vi "探头窗口-20-服务器版.vi"() -> ()   [LabVIEW 2013]
panel:
  in  "外部停止命令？":bool=TRUE
  out "引用-探头属性[]":refnum<vi>
  out "引用-监测模式？":refnum<vi>
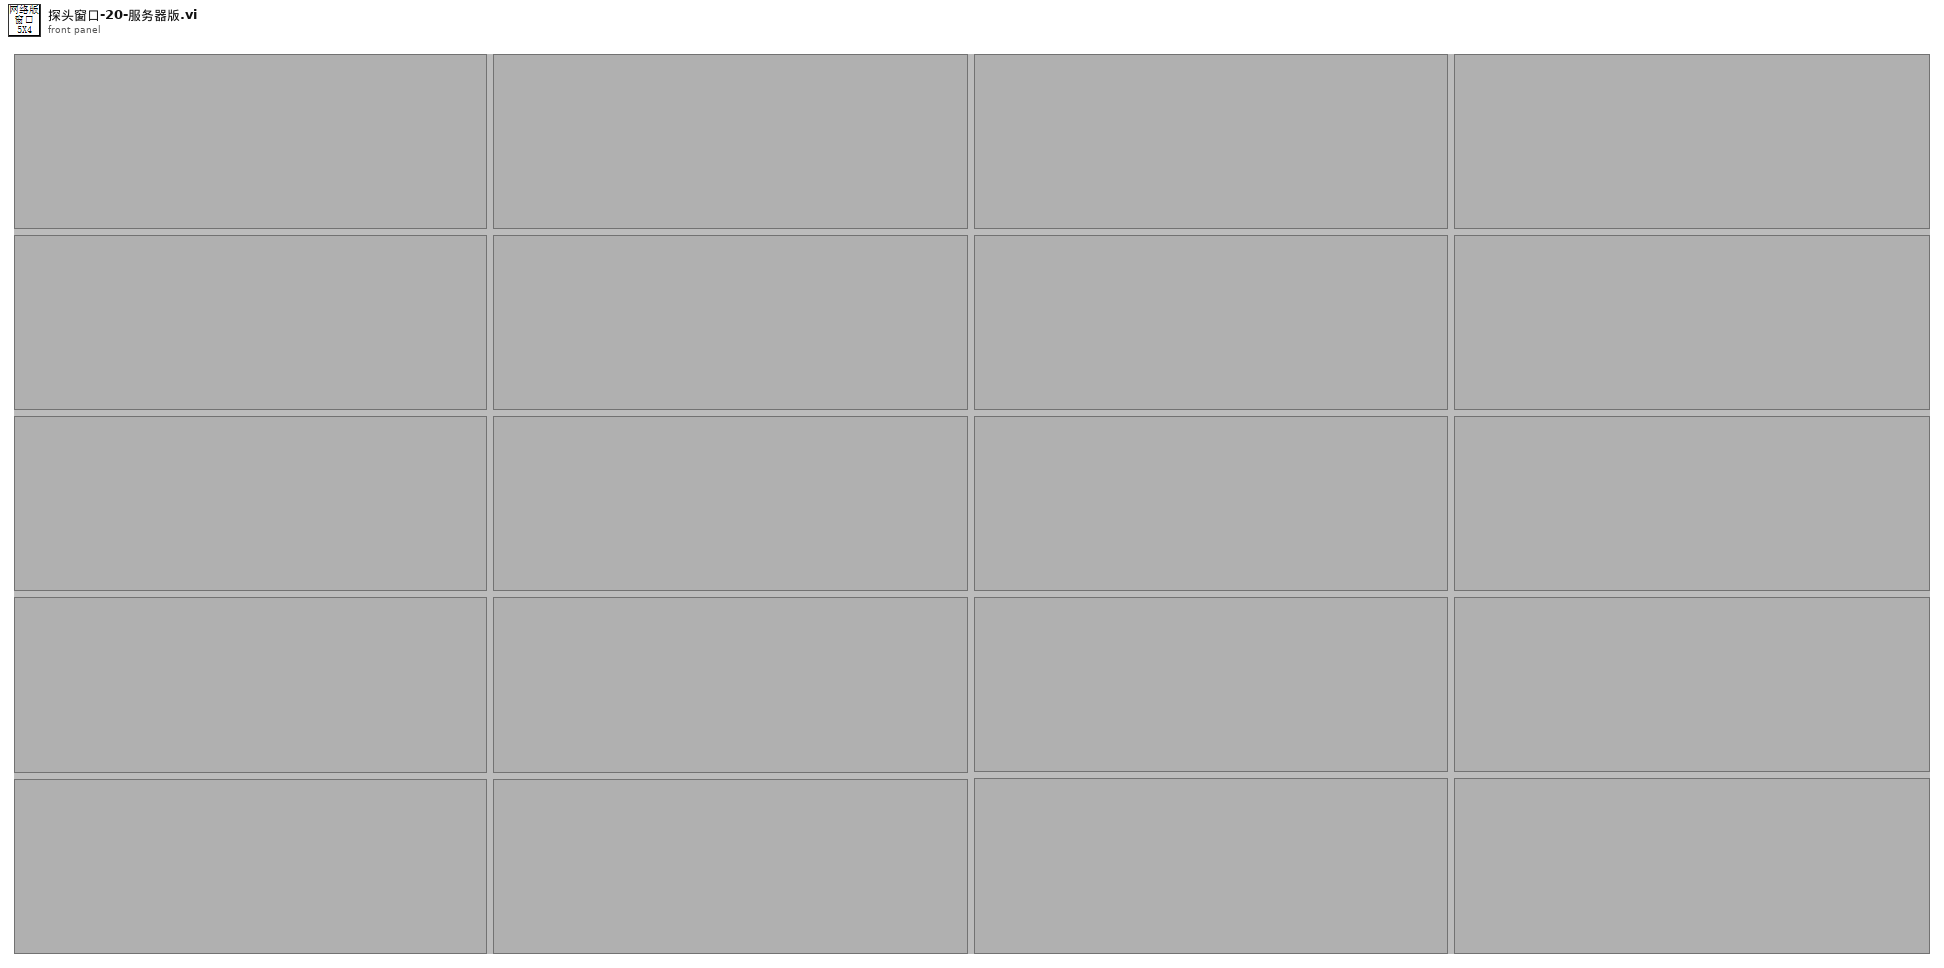
[diagram p1: front panel]
types:
  T1 = typedef "eventvkey.ctl" = enum16{"ASCII", "Enter", "Return", "Shift", "Ctrl", "Alt", "Cmd", "Opt", "Caps", "NumLock", "Clear", "Break", "Up", "Down", "Left", "Right", "Insert", "Delete", "Home", "End", "PageUp", "PageDown", "Escape", "Help", "Pause", "ScrollLock", "F1", "F2", "F3", "F4", "F5", "F6", "F7", "F8", "F9", "F10", "F11", "F12", "F13", "F14", "F15", "F16", "F17", "F18", "F19", "F20", "F21", "F22", "F23", "F24", "Play", "VolumeUp", "VolumeDown", "Mute", "Two Byte Char"}
  T2 = cluster{"探头地址与信息":cluster{"网络地址":cluster{"IP":string, "port":u16}, "探头信息":string}, "测量值":cluster{"时间":timestamp, "数值":dbl}, "限值":cluster{"限值1":dbl, "限值2":dbl}, "探头状态":enum16{"正常", "离线", "禁用", "一级报警", "二级报警"}}[]
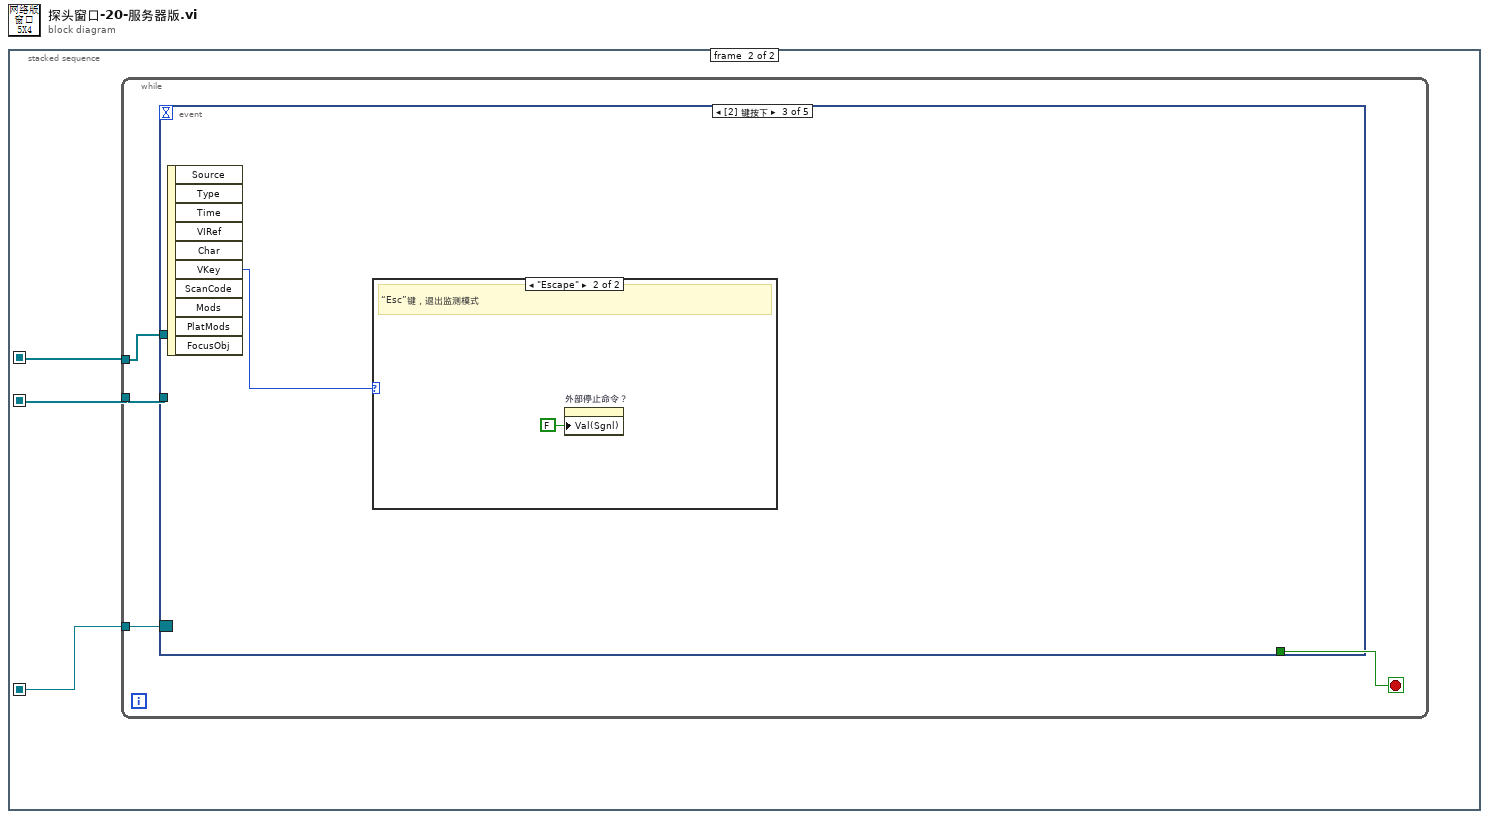
[diagram p0: block diagram]
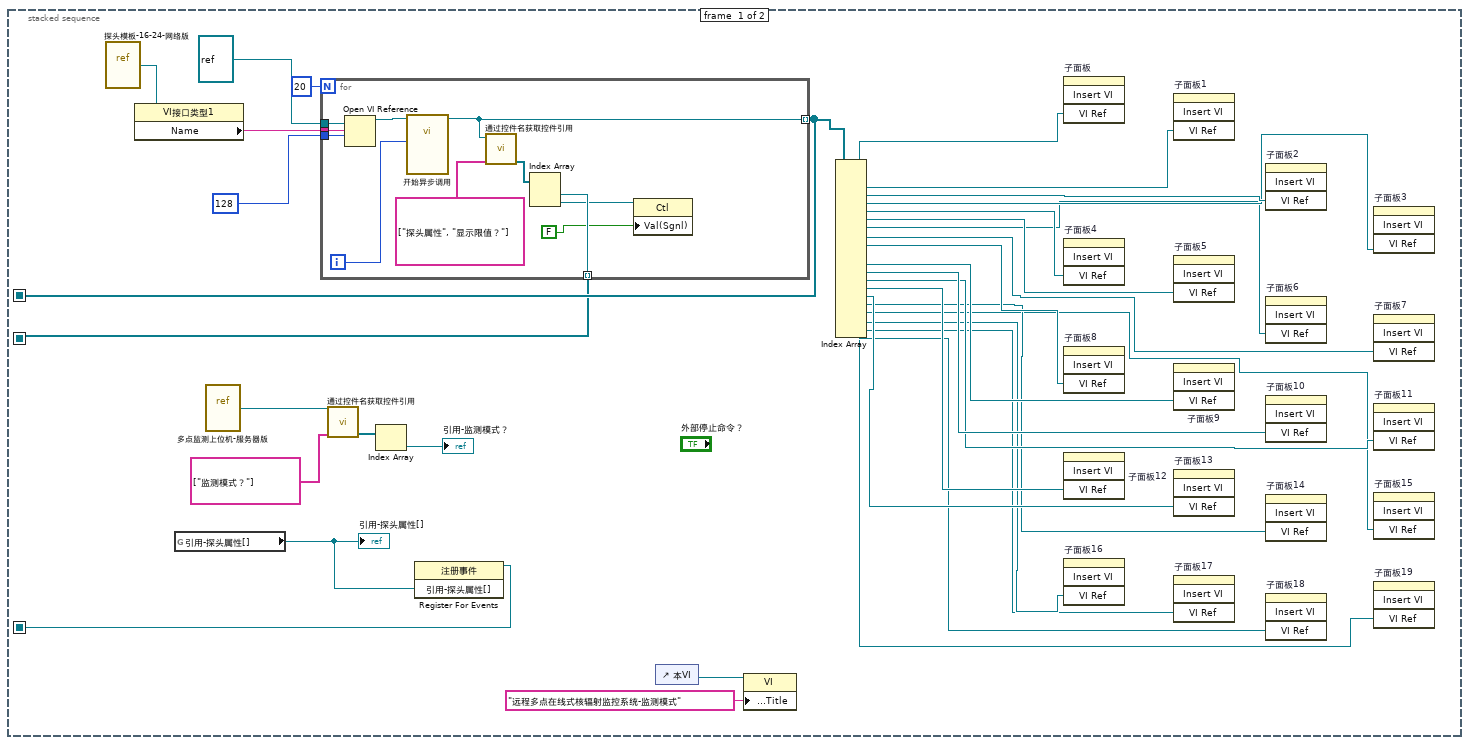
[diagram p2: hidden frame]
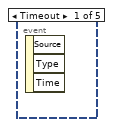
[diagram p3: hidden frame]
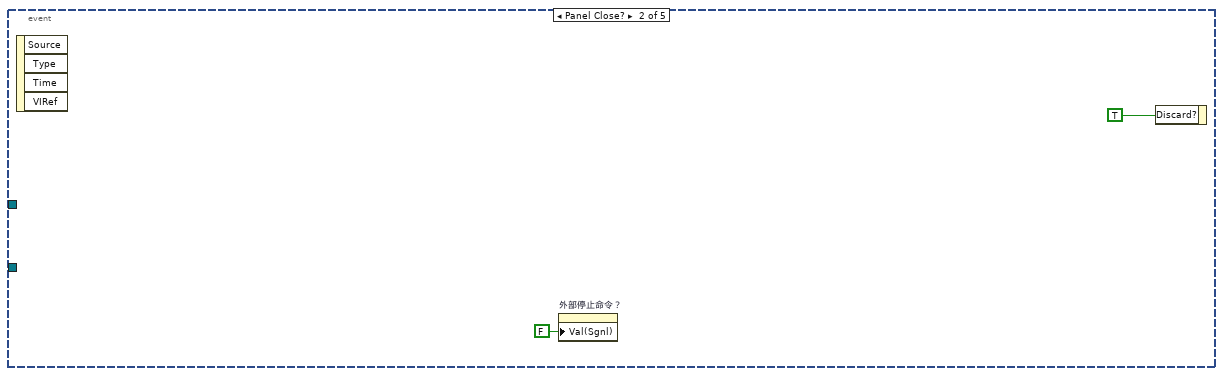
[diagram p4: hidden frame]
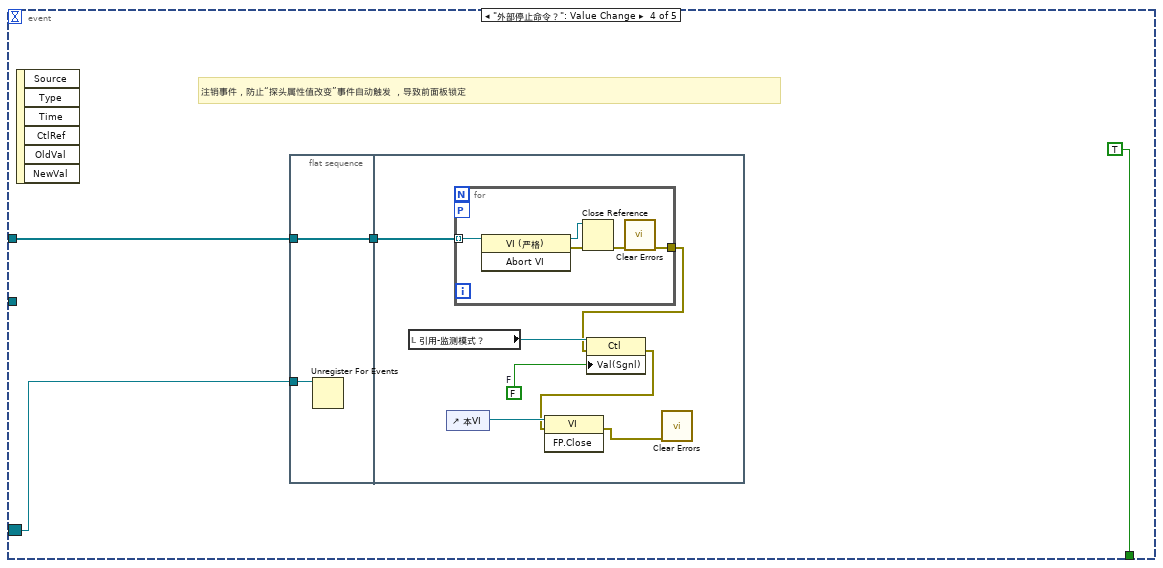
[diagram p6: hidden frame]
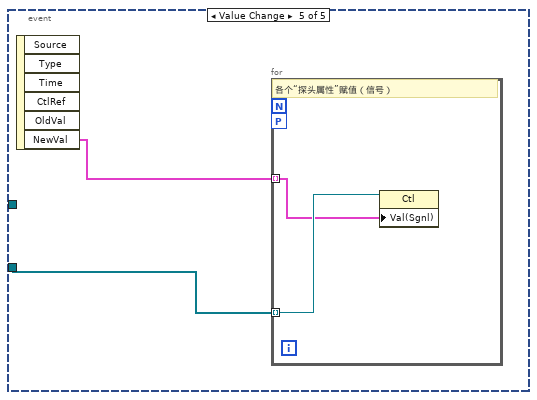
[diagram p7: hidden frame]
diagram:
  n1 = stacked-sequence {
    seq-local: [w30 _] -> [_ w49]
    seq-local: [w9 _] -> [_ w48]
    seq-local: [w3 _] -> [_ w47]
    frame #0 {
      n2 = vi-ref "探头模板-16-24-网络版.vi"() -> (w35:refnum<vi>)
      n3 = property class="VI接口类型1"(reference=w35) -> ("Name"=w34:string)  [unwired: 1 in, 2 out]
      n4 = global read "全局变量-35点监测.vi" "引用-探头属性[]"() -> (w4:refnum<vi>)
      "引用-探头属性[]" <- w4
      n5 = vi-ref "多点监测上位机-服务器版.vi"() -> (w5:refnum<vi>)
      n6 = for {
        N: 20 -> [_]
        tunnel: w34 -> [w46]
        tunnel: 128 ("选项") -> [w45]
        tunnel: refnum<vi> refnum ("类型说明符VI引用句柄（仅用于类型）") -> [w44]
        tunnel: [w39] -> w30 mode=indexing
        tunnel: [w40] -> w9 mode=indexing
        i -> [w36]
        n7 = Open VI Reference(type specifier VI Refnum (for type only)=w44, vi path=w46, options=w45) -> (vi reference=w41:refnum<vi>)  [unwired: 3 in, 1 out]
        n8 = call-by-ref "开始异步调用"(reference=w41, "探头序号"=w36) -> (reference out=w39:refnum<vi>)  [unwired: 12 in, 1 out]
        n9 = call "通过控件名获取控件引用.vi"("控件名数组"=string[] ["探头属性", "显示限值？"], "VI引用"=w39) -> ("控件引用输出"=w43:refnum<vi>[])  [unwired: 7 in, 2 out]
        n10 = Index Array(array=w43) -> (element #1=w40:refnum<vi>, element #2=w38:refnum<vi>)  [unwired: 2 in]
        n11 = property class="Ctl"(reference=w38, "Val(Sgnl)"=FALSE) -> ()  [unwired: 1 in, 2 out]
      }
      n12 = call "通过控件名获取控件引用.vi"("控件名数组"=string[] ["监测模式？"], "VI引用"=w5) -> ("控件引用输出"=w7:refnum<vi>[])  [unwired: 7 in, 2 out]
      n13 = Index Array(array=w7) -> (element=→"引用-监测模式？":refnum<vi>)  [unwired: 1 in]
      n14 = register-events(w4) -> (reference out=w3:refnum<event-registration>)  [unwired: 2 in, 1 out]
      n15 = control-ref of="本VI"() -> (w2:refnum<vi>)
      n16 = property class="VI"(reference=w2, "Front Panel.Title"="远程多点在线式核辐射监控系统-监测模式" ("前面板窗口:标题")) -> ()  [unwired: 1 in, 2 out]
      n17 = Index Array(array=w30) -> (element #1=w29:refnum<vi>, element #2=w28:refnum<vi>, element #3=w27:refnum<vi>, element #4=w26:refnum<vi>, element #5=w25:refnum<vi>, element #6=w24:refnum<vi>, element #7=w23:refnum<vi>, element #8=w22:refnum<vi>, element #9=w21:refnum<vi>, element #10=w20:refnum<vi>, element #11=w19:refnum<vi>, element #12=w18:refnum<vi>, element #13=w17:refnum<vi>, element #14=w16:refnum<vi>, element #15=w15:refnum<vi>, element #16=w14:refnum<vi>, element #17=w13:refnum<vi>, element #18=w12:refnum<vi>, element #19=w11:refnum<vi>, element #20=w10:refnum<vi>)  [unwired: 20 in]
      n18 = invoke on="子面板" class="子面板" method="Insert VI"("VI Ref"=w29) -> ()  [unwired: 3 in, 4 out]
      n19 = invoke on="子面板4" class="SubPnl" method="Insert VI"("VI Ref"=w25) -> ()  [unwired: 3 in, 4 out]
      n20 = invoke on="子面板8" class="SubPnl" method="Insert VI"("VI Ref"=w21) -> ()  [unwired: 3 in, 4 out]
      n21 = invoke on="子面板12" class="SubPnl" method="Insert VI"("VI Ref"=w17) -> ()  [unwired: 3 in, 4 out]
      n22 = invoke on="子面板16" class="SubPnl" method="Insert VI"("VI Ref"=w13) -> ()  [unwired: 3 in, 4 out]
      n23 = invoke on="子面板1" class="SubPnl" method="Insert VI"("VI Ref"=w28) -> ()  [unwired: 3 in, 4 out]
      n24 = invoke on="子面板5" class="SubPnl" method="Insert VI"("VI Ref"=w24) -> ()  [unwired: 3 in, 4 out]
      n25 = invoke on="子面板9" class="SubPnl" method="Insert VI"("VI Ref"=w20) -> ()  [unwired: 3 in, 4 out]
      n26 = invoke on="子面板13" class="SubPnl" method="Insert VI"("VI Ref"=w16) -> ()  [unwired: 3 in, 4 out]
      n27 = invoke on="子面板17" class="SubPnl" method="Insert VI"("VI Ref"=w12) -> ()  [unwired: 3 in, 4 out]
      n28 = invoke on="子面板2" class="SubPnl" method="Insert VI"("VI Ref"=w27) -> ()  [unwired: 3 in, 4 out]
      n29 = invoke on="子面板6" class="SubPnl" method="Insert VI"("VI Ref"=w23) -> ()  [unwired: 3 in, 4 out]
      n30 = invoke on="子面板10" class="SubPnl" method="Insert VI"("VI Ref"=w19) -> ()  [unwired: 3 in, 4 out]
      n31 = invoke on="子面板14" class="SubPnl" method="Insert VI"("VI Ref"=w15) -> ()  [unwired: 3 in, 4 out]
      n32 = invoke on="子面板18" class="SubPnl" method="Insert VI"("VI Ref"=w11) -> ()  [unwired: 3 in, 4 out]
      n33 = invoke on="子面板3" class="SubPnl" method="Insert VI"("VI Ref"=w26) -> ()  [unwired: 3 in, 4 out]
      n34 = invoke on="子面板7" class="SubPnl" method="Insert VI"("VI Ref"=w22) -> ()  [unwired: 3 in, 4 out]
      n35 = invoke on="子面板11" class="SubPnl" method="Insert VI"("VI Ref"=w18) -> ()  [unwired: 3 in, 4 out]
      n36 = invoke on="子面板15" class="SubPnl" method="Insert VI"("VI Ref"=w14) -> ()  [unwired: 3 in, 4 out]
      n37 = invoke on="子面板19" class="SubPnl" method="Insert VI"("VI Ref"=w10) -> ()  [unwired: 3 in, 4 out]
    }
    frame #1 {
      n38 = while {
        tunnel: w49 -> [w52]
        tunnel: w48 -> [w51]
        tunnel: w47 -> [w50]
        stop <- w53 stop-if-true
        n39 = event shown="[2] 键按下" {
          selector: w50 -> [_ _ _ w58 _]
          dyn-events: _ -> [_ _ _ _ _]
          timeout: _ -> [_ _ _ _ _]
          tunnel: [_ _ _ TRUE ("放弃？") _] -> w53
          tunnel: w52 -> [_ _ _ w60 _]
          tunnel: w51 -> [_ _ _ _ w76]
          event Timeout {
            n40 = event-data() -> ()  [unwired: 1 in, 3 out]
          }
          event Panel Close? {
            n41 = event-data() -> ()  [unwired: 1 in, 4 out]
            n42 = property on="外部停止命令？" class="Bool (严格)"("Val(Sgnl)"=FALSE ("值(信号)")) -> ()  [unwired: 2 in, 2 out]
            n43 = event-data("Discard?"=TRUE ("放弃？")) -> ()  [unwired: 1 in, 1 out]
          }
          event Key Down {
            n44 = event-data() -> ("VKey"=w56:T1)  [unwired: 1 in, 9 out]
            n45 = case shown="\"Escape\"" w56 {
              frame "ASCII", Default {
              }
              frame "Escape" {
                # "“Esc”键，退出监测模式"
                n46 = property on="外部停止命令？" class="Bool (严格)"("Val(Sgnl)"=FALSE ("值(信号)")) -> ()  [unwired: 2 in, 2 out]
              }
            }
          }
          event "外部停止命令？": Value Change {
            # "注销事件，防止“探头属性值改变”事件自动触发 ，导致前面板锁定"
            n47 = event-data() -> ()  [unwired: 1 in, 6 out]
            n48 = flat-sequence {
              tunnel: w60 -> [w63]
              tunnel: [w63] -> w59
              tunnel: w58 -> [w62]
              tunnel: w59 -> [w70]
              frame #0 {
                n49 = Unregister For Events(event registration refnum=w62) -> ()  [unwired: 1 in, 1 out]
              }
              frame #1 {
                w69 = FALSE  # F
                n50 = local read "引用-监测模式？"() -> (w68:refnum<vi>)
                n51 = control-ref of="本VI"() -> (w67:refnum<vi>)
                n52 = for {
                  tunnel: w70 -> [w75] mode=indexing
                  workers-P: _ -> [_]
                  tunnel: [w71] -> w66
                  n53 = invoke class="VI (严格)" method="Abort VI"(reference=w75) -> (reference out=w73:refnum<vi>, error out=w74:errorcluster)  [unwired: 2 in, 1 out]
                  n54 = Close Reference(reference=w73, error in (no error)=w74) -> (error out=w72:errorcluster)
                  n55 = call <vilib>:"Clear Errors.vi"("error in (no error)"=w72) -> ("error out"=w71:errorcluster)  [unwired: 6 in]
                }
                n56 = property class="Ctl"(reference=w68, error in=w66, "Val(Sgnl)"=w69) -> (error out=w65:errorcluster)  [unwired: 1 out]
                n57 = invoke class="VI" method="FP.Close"(reference=w67, error in=w65) -> (error out=w64:errorcluster)  [unwired: 1 in, 2 out]
                n58 = call <vilib>:"Clear Errors.vi"("error in (no error)"=w64) -> ()  [unwired: 6 in, 1 out]
              }
            }
          }
          event Value Change {
            n59 = event-data() -> ("NewVal"=w77:T2)  [unwired: 1 in, 5 out]
            n60 = for {
              workers-P: _ -> [_]
              tunnel: w76 -> [w79] mode=indexing
              tunnel: w77 -> [w78] mode=indexing
              # "各个“探头属性”赋值（信号）"
              n61 = property class="Ctl"(reference=w79, "Val(Sgnl)"=w78) -> ()  [unwired: 1 in, 2 out]
            }
          }
        }
      }
    }
  }
